vi "RT Driver VI.vi"(6 "Device Clock":string, 9 "Device Inputs FIFO":refnum<k33>, 10 "Device Outputs FIFO":refnum<k33>, 11 "Device Reference":T4 format="%.0x") -> ()   [LabVIEW 2017, in "ALMA_10201-10401_O2SensorSim Engine.lvlib"]
uses:
  ALMA_10201-10401_O2SensorSim Engine.lvlib
  <vilib>/NI Veristand/Custom Device API/Custom Device Item Ref.ctl
  Par.ctl
  LambdaType.ctl
  Sensor_used.ctl
  <vilib>/NI Veristand/Custom Device API/Custom Device Channel Type.ctl
  <vilib>/Platform/TimedLoop/XDataNode/timing_clust.ctl
  <vilib>/Platform/TimedLoop/XDataNode/nitl_modes.ctl
  <vilib>/Platform/TimedLoop/XDataNode/wakeup.ctl
  <vilib>/NI Veristand/Custom Device API/Message Response (String).ctl
  <vilib>/NI Veristand/Custom Device API/Message Response (Byte Array).ctl
  <vilib>/NI Veristand/Custom Device API/Get Item Property (String).vi
  <vilib>/SLSC/Initialize Session with Devices.vi
  <vilib>/SLSC/Close Session.vi
  <vilib>/Platform/TimedLoop/XDataNode/XDataNode.xnode
  <vilib>/NI Veristand/Custom Device API/Custom Device API.lvlib
  <vilib>/NI Veristand/Custom Device Tools/Custom Device Utility Library/Custom Device Utility Library.lvlib
  <vilib>/Platform/TimedLoop/XDataNode/XDNodeRunTimeDep.lvlib
  <vilib>/SLSC/SLSC.lvlib
  System Explorer/SLSC CD API/SLSC CD Engine/SLSC CD Engine.lvlib
panel:
  in  "SensorUsed":T1
  out "Device Session":refnum<k21>
  in  "par 2":T2={"Loop time"={"Loop Rate"=0, "Processor"=0}, "COM"={"COM IP"="0.0.0.0", "COM port"=1, "Local port"=0, "Next_IP 1"=0, "Next_IP 2"=0, "Next_IP 3"=0, "Next_IP 4"=0}, "O2Sensor1"={"Lambda"={"LSU4.2 Lambda"=[], "LSU4.2 Ip"=[], "LSU4.9 Lambda"=[], "LSU4.9 Ip"=[], "LZA03 Lambda"=[], "LZA03 Ip"=[], "LZA08 Lambda"=[], "LZA08 Ip"=[], "Custom Lambda"=[], "Custom Ip"=[]}, "Temp"={"LSU4.2 Temp"=[], "LSU4.2 Ohm"=[], "LSU4.9 Temp"=[], "LSU4.9 Ohm"=[], "LZA03 Temp"=[], "LZA03 Ohm"=[], "LZA08 Temp"=[], "LZA08 Ohm"=[], "Custom Temp"=[], "Custom Ohm"=[]}, "Lambda Type"=0, "PID"={"Ki"=0.0, "Kp"=0.0, "Kd"=0.0, "FeedFW"=0.0}}, "O2Sensor2"={"Lambda"={"LSU4.2 Lambda"=[], "LSU4.2 Ip"=[], "LSU4.9 Lambda"=[], "LSU4.9 Ip"=[], "LZA03 Lambda"=[], "LZA03 Ip"=[], "LZA08 Lambda"=[], "LZA08 Ip"=[], "Custom Lambda"=[], "Custom Ip"=[]}, "Temp"={"LSU4.2 Temp"=[], "LSU4.2 Ohm"=[], "LSU4.9 Temp"=[], "LSU4.9 Ohm"=[], "LZA03 Temp"=[], "LZA03 Ohm"=[], "LZA08 Temp"=[], "LZA08 Ohm"=[], "Custom Temp"=[], "Custom Ohm"=[]}, "Lambda Type"=0, "PID"={"Ki"=0.0, "Kp"=0.0, "Kd"=0.0, "FeedFW"=0.0}}, "O2Sensor3"={"Lambda"={"LSU4.2 Lambda"=[], "LSU4.2 Ip"=[], "LSU4.9 Lambda"=[], "LSU4.9 Ip"=[], "LZA03 Lambda"=[], "LZA03 Ip"=[], "LZA08 Lambda"=[], "LZA08 Ip"=[], "Custom Lambda"=[], "Custom Ip"=[]}, "Temp"={"LSU4.2 Temp"=[], "LSU4.2 Ohm"=[], "LSU4.9 Temp"=[], "LSU4.9 Ohm"=[], "LZA03 Temp"=[], "LZA03 Ohm"=[], "LZA08 Temp"=[], "LZA08 Ohm"=[], "Custom Temp"=[], "Custom Ohm"=[]}, "Lambda Type"=0, "PID"={"Ki"=0.0, "Kp"=0.0, "Kd"=0.0, "FeedFW"=0.0}}, "O2Sensor4"={"Lambda"={"LSU4.2 Lambda"=[], "LSU4.2 Ip"=[], "LSU4.9 Lambda"=[], "LSU4.9 Ip"=[], "LZA03 Lambda"=[], "LZA03 Ip"=[], "LZA08 Lambda"=[], "LZA08 Ip"=[], "Custom Lambda"=[], "Custom Ip"=[]}, "Temp"={"LSU4.2 Temp"=[], "LSU4.2 Ohm"=[], "LSU4.9 Temp"=[], "LSU4.9 Ohm"=[], "LZA03 Temp"=[], "LZA03 Ohm"=[], "LZA08 Temp"=[], "LZA08 Ohm"=[], "Custom Temp"=[], "Custom Ohm"=[]}, "Lambda Type"=0, "PID"={"Ki"=0.0, "Kp"=0.0, "Kd"=0.0, "FeedFW"=0.0}}, "Board"=0, "Mode"=enum."SLSC Mode", "vendor.Num"=4141, "product.Num"=0} {"Board" items=["O2Sim_2ch", "O2Sim_4ch"]; "O2Sensor4"."Lambda Type" items=["LSU4.2", "LSU4.9", "LZA03", "LZA08", "Custom", "[mA]"]; "O2Sensor3"."Lambda Type" items=["LSU4.2", "LSU4.9", "LZA03", "LZA08", "Custom", "[mA]"]; "O2Sensor2"."Lambda Type" items=["LSU4.2", "LSU4.9", "LZA03", "LZA08", "Custom", "[mA]"]; "O2Sensor1"."Lambda Type" items=["LSU4.2", "LSU4.9", "LZA03", "LZA08", "Custom", "[mA]"]}
  in  "Initialization Status Notifier":refnum<notifier>
  in  "Status Notifier":refnum<notifier>
  # "Custom Device Template\nv1.0"
  # "Use this template as a starting point for creating a custom device code module. The input controls shown here are specially named controls that the system will use to provide the device loop with data. The controls are not required for the device loop to run. For instance, if the device doesn't produce any output data, then you don't need the Device Outputs FIFO control. If you do use these controls, however, they need to have these exact names to be functional."
  # "The optional status notifier element is used to notify the RT engine of the last state of the custom device, and to indicate the device has completed execution. If this control is not used, a default No Error value is returned to the system when the device finishes execution.\n\nNote: This error state is not checked until the system shuts down. Use an output status channel to send more immediate status values to the system."
  # "This optional input can be used to send the VeriStand Engine the final status of the custom device initalization process. If this control exists on the custom device front panel, the VeriStand Engine will wait for a status update before starting up. If the custom device reports an error, that will abort the execution of the current configuration in the VeriStand Engine.\n\nThis control can be deleted if the custom device does not need to send the initialization status update."
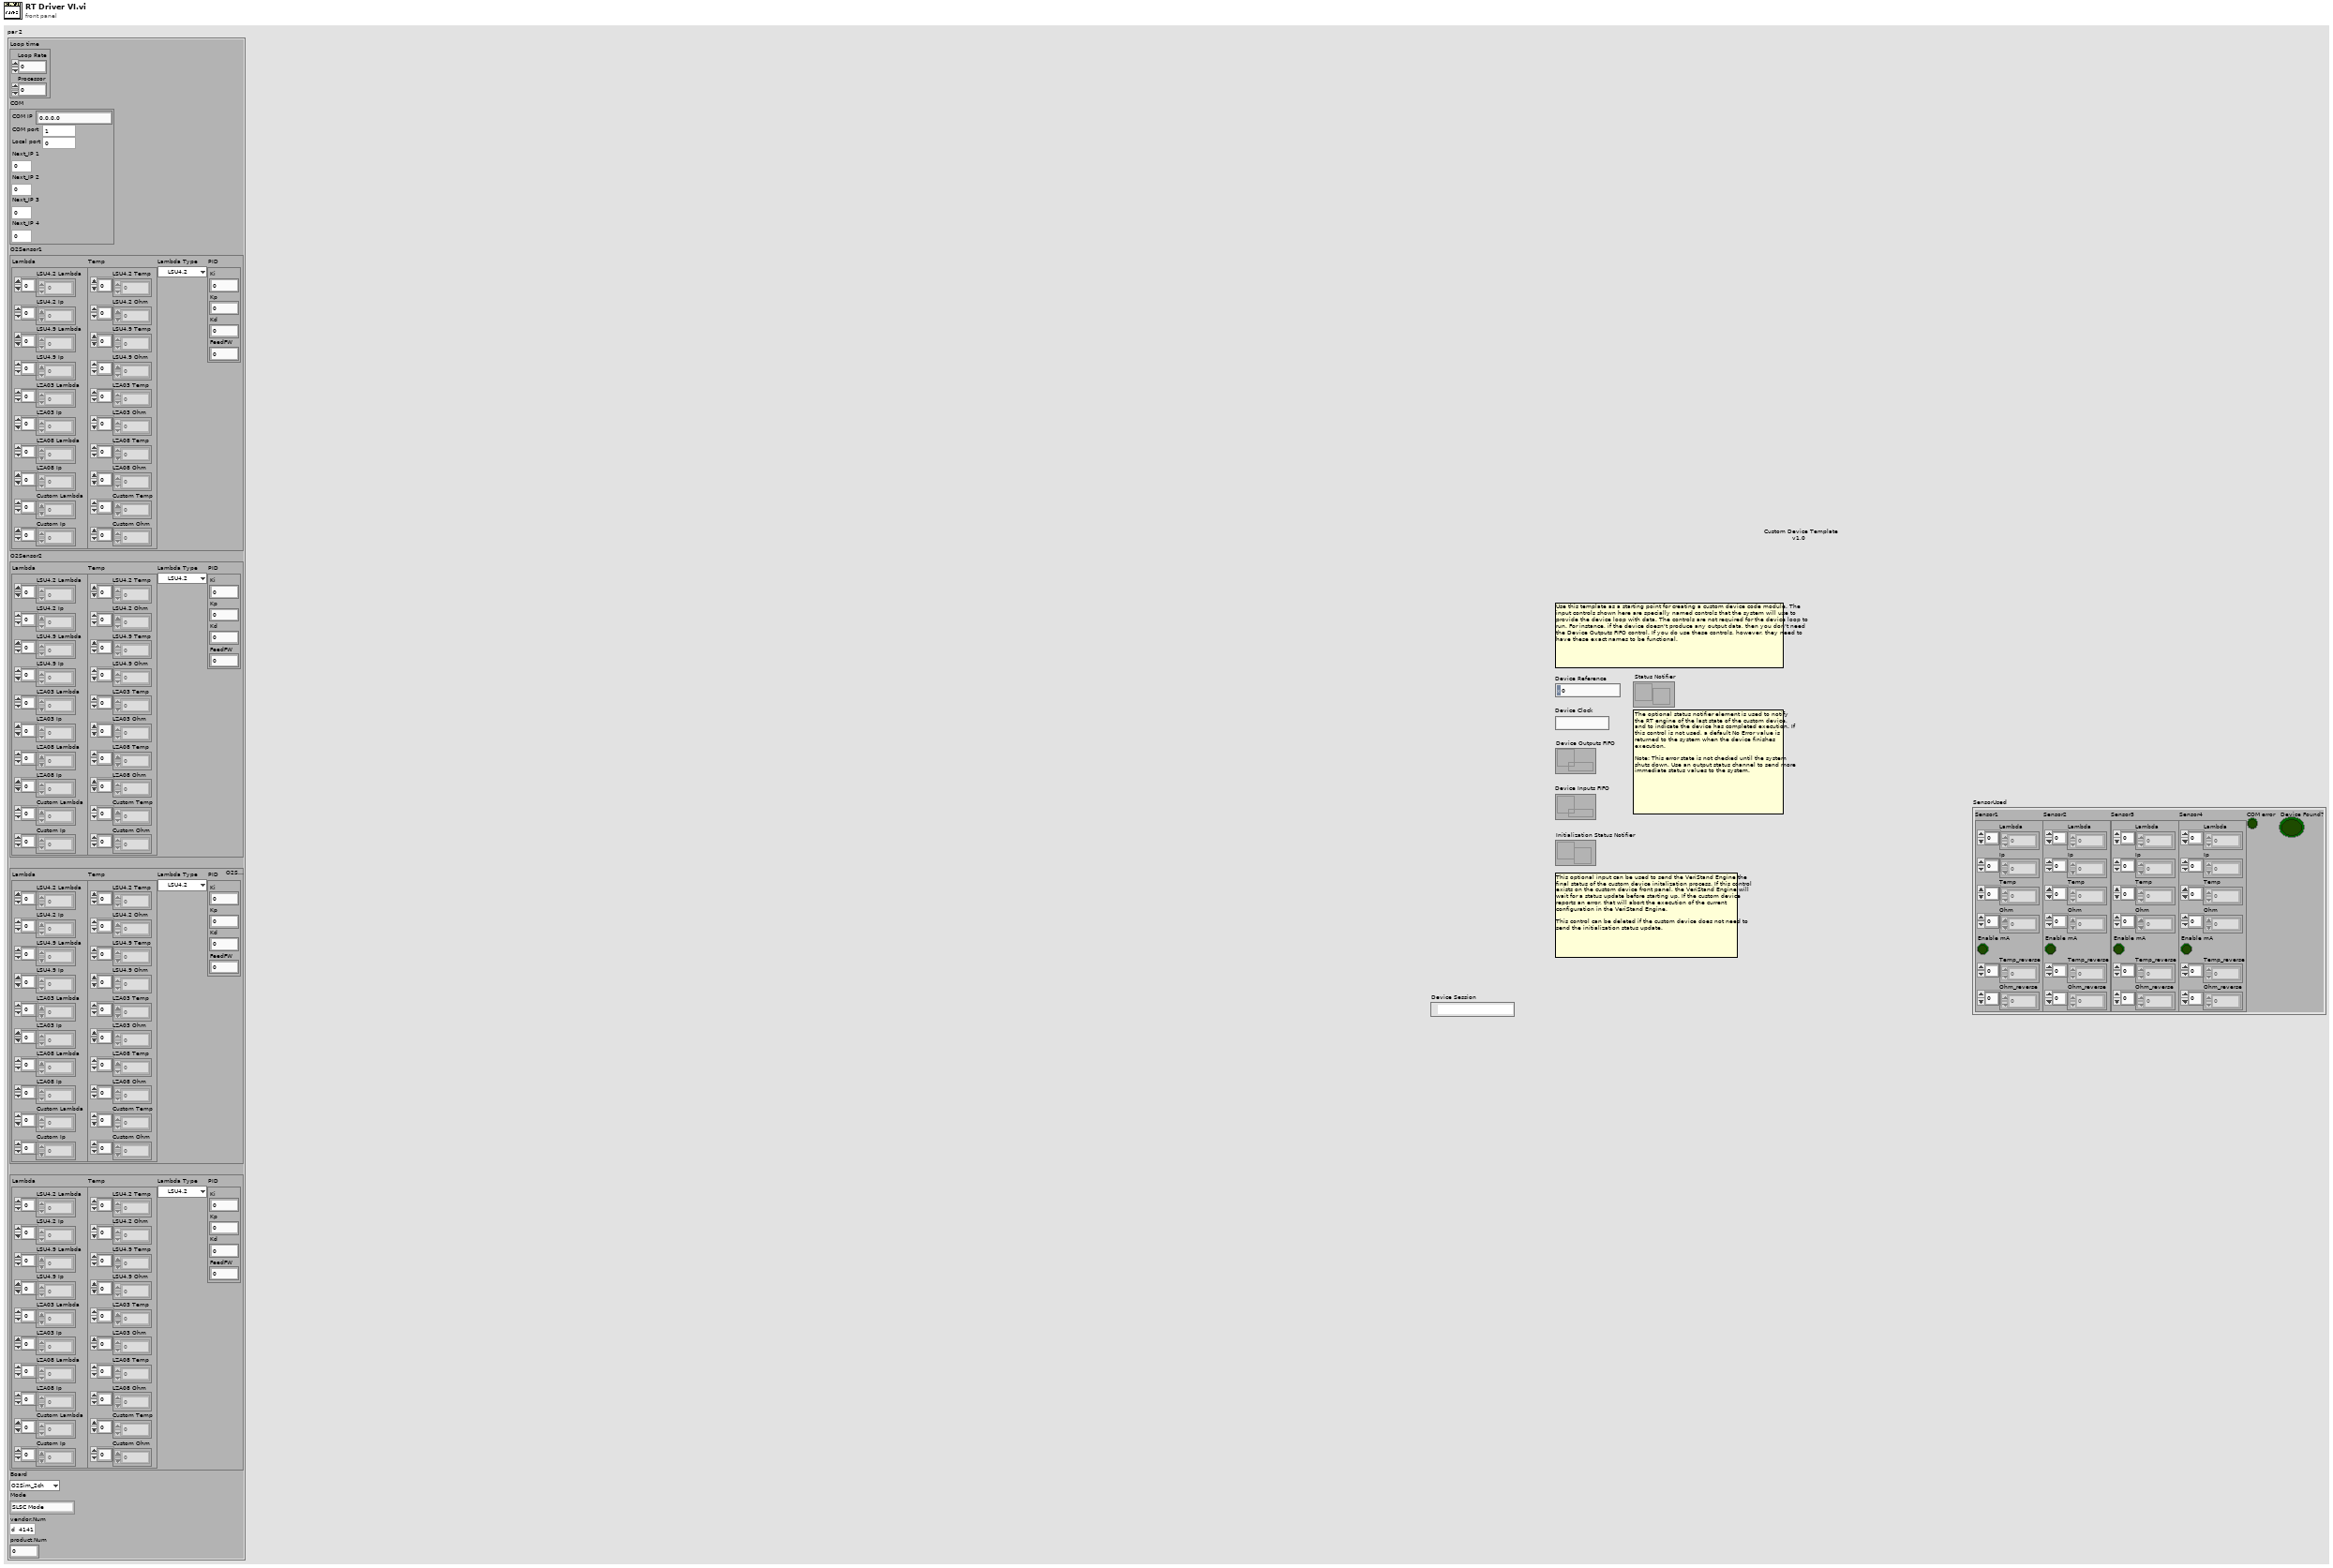
[diagram p1: front panel]
types:
  T1 = typedef "ALMA_10201-10401_O2SensorSim Engine.lvlib/Sensor_used.ctl" = cluster{"Sensor1":cluster{"Lambda":dbl[], "Ip":dbl[], "Temp":dbl[], "Ohm":dbl[], "Enable mA":bool, "Temp_reverse":dbl[], "Ohm_reverse":dbl[]}, "Sensor2":cluster{"Lambda":dbl[], "Ip":dbl[], "Temp":dbl[], "Ohm":dbl[], "Enable mA":bool, "Temp_reverse":dbl[], "Ohm_reverse":dbl[]}, "Sensor3":cluster{"Lambda":dbl[], "Ip":dbl[], "Temp":dbl[], "Ohm":dbl[], "Enable mA":bool, "Temp_reverse":dbl[], "Ohm_reverse":dbl[]}, "Sensor4":cluster{"Lambda":dbl[], "Ip":dbl[], "Temp":dbl[], "Ohm":dbl[], "Enable mA":bool, "Temp_reverse":dbl[], "Ohm_reverse":dbl[]}, "COM error":bool, "Device Found?":bool}
  T2 = typedef "Par.ctl" = cluster{"Loop time":cluster{"Loop Rate":i64, "Processor":i32}, "COM":cluster{"COM IP":string, "COM port":u64, "Local port":u64, "Next_IP 1":u32, "Next_IP 2":u32, "Next_IP 3":u32, "Next_IP 4":u32}, "O2Sensor1":cluster{"Lambda":cluster{"LSU4.2 Lambda":dbl[], "LSU4.2 Ip":dbl[], "LSU4.9 Lambda":dbl[], "LSU4.9 Ip":dbl[], "LZA03 Lambda":dbl[], "LZA03 Ip":dbl[], "LZA08 Lambda":dbl[], "LZA08 Ip":dbl[], "Custom Lambda":dbl[], "Custom Ip":dbl[]}, "Temp":cluster{"LSU4.2 Temp":dbl[], "LSU4.2 Ohm":dbl[], "LSU4.9 Temp":dbl[], "LSU4.9 Ohm":dbl[], "LZA03 Temp":dbl[], "LZA03 Ohm":dbl[], "LZA08 Temp":dbl[], "LZA08 Ohm":dbl[], "Custom Temp":dbl[], "Custom Ohm":dbl[]}, "Lambda Type":T3, "PID":cluster{"Ki":dbl, "Kp":dbl, "Kd":dbl, "FeedFW":dbl}}, "O2Sensor2":cluster{"Lambda":cluster{"LSU4.2 Lambda":dbl[], "LSU4.2 Ip":dbl[], "LSU4.9 Lambda":dbl[], "LSU4.9 Ip":dbl[], "LZA03 Lambda":dbl[], "LZA03 Ip":dbl[], "LZA08 Lambda":dbl[], "LZA08 Ip":dbl[], "Custom Lambda":dbl[], "Custom Ip":dbl[]}, "Temp":cluster{"LSU4.2 Temp":dbl[], "LSU4.2 Ohm":dbl[], "LSU4.9 Temp":dbl[], "LSU4.9 Ohm":dbl[], "LZA03 Temp":dbl[], "LZA03 Ohm":dbl[], "LZA08 Temp":dbl[], "LZA08 Ohm":dbl[], "Custom Temp":dbl[], "Custom Ohm":dbl[]}, "Lambda Type":T3, "PID":cluster{"Ki":dbl, "Kp":dbl, "Kd":dbl, "FeedFW":dbl}}, "O2Sensor3":cluster{"Lambda":cluster{"LSU4.2 Lambda":dbl[], "LSU4.2 Ip":dbl[], "LSU4.9 Lambda":dbl[], "LSU4.9 Ip":dbl[], "LZA03 Lambda":dbl[], "LZA03 Ip":dbl[], "LZA08 Lambda":dbl[], "LZA08 Ip":dbl[], "Custom Lambda":dbl[], "Custom Ip":dbl[]}, "Temp":cluster{"LSU4.2 Temp":dbl[], "LSU4.2 Ohm":dbl[], "LSU4.9 Temp":dbl[], "LSU4.9 Ohm":dbl[], "LZA03 Temp":dbl[], "LZA03 Ohm":dbl[], "LZA08 Temp":dbl[], "LZA08 Ohm":dbl[], "Custom Temp":dbl[], "Custom Ohm":dbl[]}, "Lambda Type":T3, "PID":cluster{"Ki":dbl, "Kp":dbl, "Kd":dbl, "FeedFW":dbl}}, "O2Sensor4":cluster{"Lambda":cluster{"LSU4.2 Lambda":dbl[], "LSU4.2 Ip":dbl[], "LSU4.9 Lambda":dbl[], "LSU4.9 Ip":dbl[], "LZA03 Lambda":dbl[], "LZA03 Ip":dbl[], "LZA08 Lambda":dbl[], "LZA08 Ip":dbl[], "Custom Lambda":dbl[], "Custom Ip":dbl[]}, "Temp":cluster{"LSU4.2 Temp":dbl[], "LSU4.2 Ohm":dbl[], "LSU4.9 Temp":dbl[], "LSU4.9 Ohm":dbl[], "LZA03 Temp":dbl[], "LZA03 Ohm":dbl[], "LZA08 Temp":dbl[], "LZA08 Ohm":dbl[], "Custom Temp":dbl[], "Custom Ohm":dbl[]}, "Lambda Type":T3, "PID":cluster{"Ki":dbl, "Kp":dbl, "Kd":dbl, "FeedFW":dbl}}, "Board":u16, "Mode":enum16{"SLSC Mode", "ANALOG Mode"}, "vendor.Num":u32, "product.Num":u32}
  T3 = typedef "LambdaType.ctl" = u16
  T4 = typedef "Custom Device API.lvlib/Custom Device Item Ref.ctl" = u64
  T5 = typedef "Custom Device API.lvlib/Custom Device Channel Type.ctl" = enum16{"Input", "Output"}
  T6 = cluster{"Lambda":cluster{"LSU4.2 Lambda":dbl[], "LSU4.2 Ip":dbl[], "LSU4.9 Lambda":dbl[], "LSU4.9 Ip":dbl[], "LZA03 Lambda":dbl[], "LZA03 Ip":dbl[], "LZA08 Lambda":dbl[], "LZA08 Ip":dbl[], "Custom Lambda":dbl[], "Custom Ip":dbl[]}, "Temp":cluster{"LSU4.2 Temp":dbl[], "LSU4.2 Ohm":dbl[], "LSU4.9 Temp":dbl[], "LSU4.9 Ohm":dbl[], "LZA03 Temp":dbl[], "LZA03 Ohm":dbl[], "LZA08 Temp":dbl[], "LZA08 Ohm":dbl[], "Custom Temp":dbl[], "Custom Ohm":dbl[]}, "Lambda Type":T3, "PID":cluster{"Ki":dbl, "Kp":dbl, "Kd":dbl, "FeedFW":dbl}}
  T7 = cluster{"Lambda":cluster{"LSU4.2 Lambda":dbl[], "LSU4.2 Ip":dbl[], "LSU4.9 Lambda":dbl[], "LSU4.9 Ip":dbl[], "LZA03 Lambda":dbl[], "LZA03 Ip":dbl[], "LZA08 Lambda":dbl[], "LZA08 Ip":dbl[], "Custom Lambda":dbl[], "Custom Ip":dbl[]}, "Temp":cluster{"LSU4.2 Temp":dbl[], "LSU4.2 Ohm":dbl[], "LSU4.9 Temp":dbl[], "LSU4.9 Ohm":dbl[], "LZA03 Temp":dbl[], "LZA03 Ohm":dbl[], "LZA08 Temp":dbl[], "LZA08 Ohm":dbl[], "Custom Temp":dbl[], "Custom Ohm":dbl[]}, "Lambda Type":T3, "PID":cluster{"Ki":dbl, "Kp":dbl, "Kd":dbl, "FeedFW":dbl}}[]
  T8 = typedef "Custom Device API.lvlib/Custom Device Engine Event Ref.ctl" = refnum<event-registration>
  T9 = cluster{"Custom Lambda":dbl[], "Custom Lambda":dbl[], "Custom Lambda":dbl[], "Custom Lambda":dbl[], bool, "Custom Lambda":dbl[], "Custom Lambda":dbl[]}
  T10 = typedef "XDNodeRunTimeDep.lvlib/timing_clust.ctl" = cluster{"Expected End [f-1]":u64, "Actual End [f-1]":u64, "Finished Late? [f-1]":bool, "Expected End [i-1]":u64, "Actual End [i-1]":u64, "Finished Late? [i-1]":bool, "Expected Start [i]":u64, "Actual Start [i]":u64, "Expected Start [f]":u64, "Actual Start [f]":u64, "Source Name":string, "Structure Name":string, "Period":i64, "Deadline":i64, "Offset":i64, "Start":i64, "Priority":i32, "Timeout":i32, "Mode":T11, "Wakeup Reason":T12, "Error":errorcluster, "Source Type":string, "Secondary Source Type":string, "Global End Time":u64, "Global Start Time":u64, "Frame Duration":u64, "Iteration Duration":u64, "Assigned CPU":i32, "I/O Scan Engine Mode":u32}
  T11 = typedef "XDNodeRunTimeDep.lvlib/nitl_modes.ctl" = enum32{"No Change", "Process missed periods, maintain original phase", "Discard missed periods, maintain original phase", "Process missed periods, ignore original phase", "Discard missed periods, ignore original phase"}
  T12 = typedef "XDNodeRunTimeDep.lvlib/wakeup.ctl" = enum32{"Normal", "Aborted", "Asynchronous wakeup", "Timing source error", "Timed loop error", "Timeout"}
  T13 = typedef "Custom Device API.lvlib/Message Response (String).ctl" = cluster{"Response":string, "Error":errorcluster}
  T14 = typedef "Custom Device API.lvlib/Message Response (Byte Array).ctl" = cluster{"Response":u8[], "Error":errorcluster}
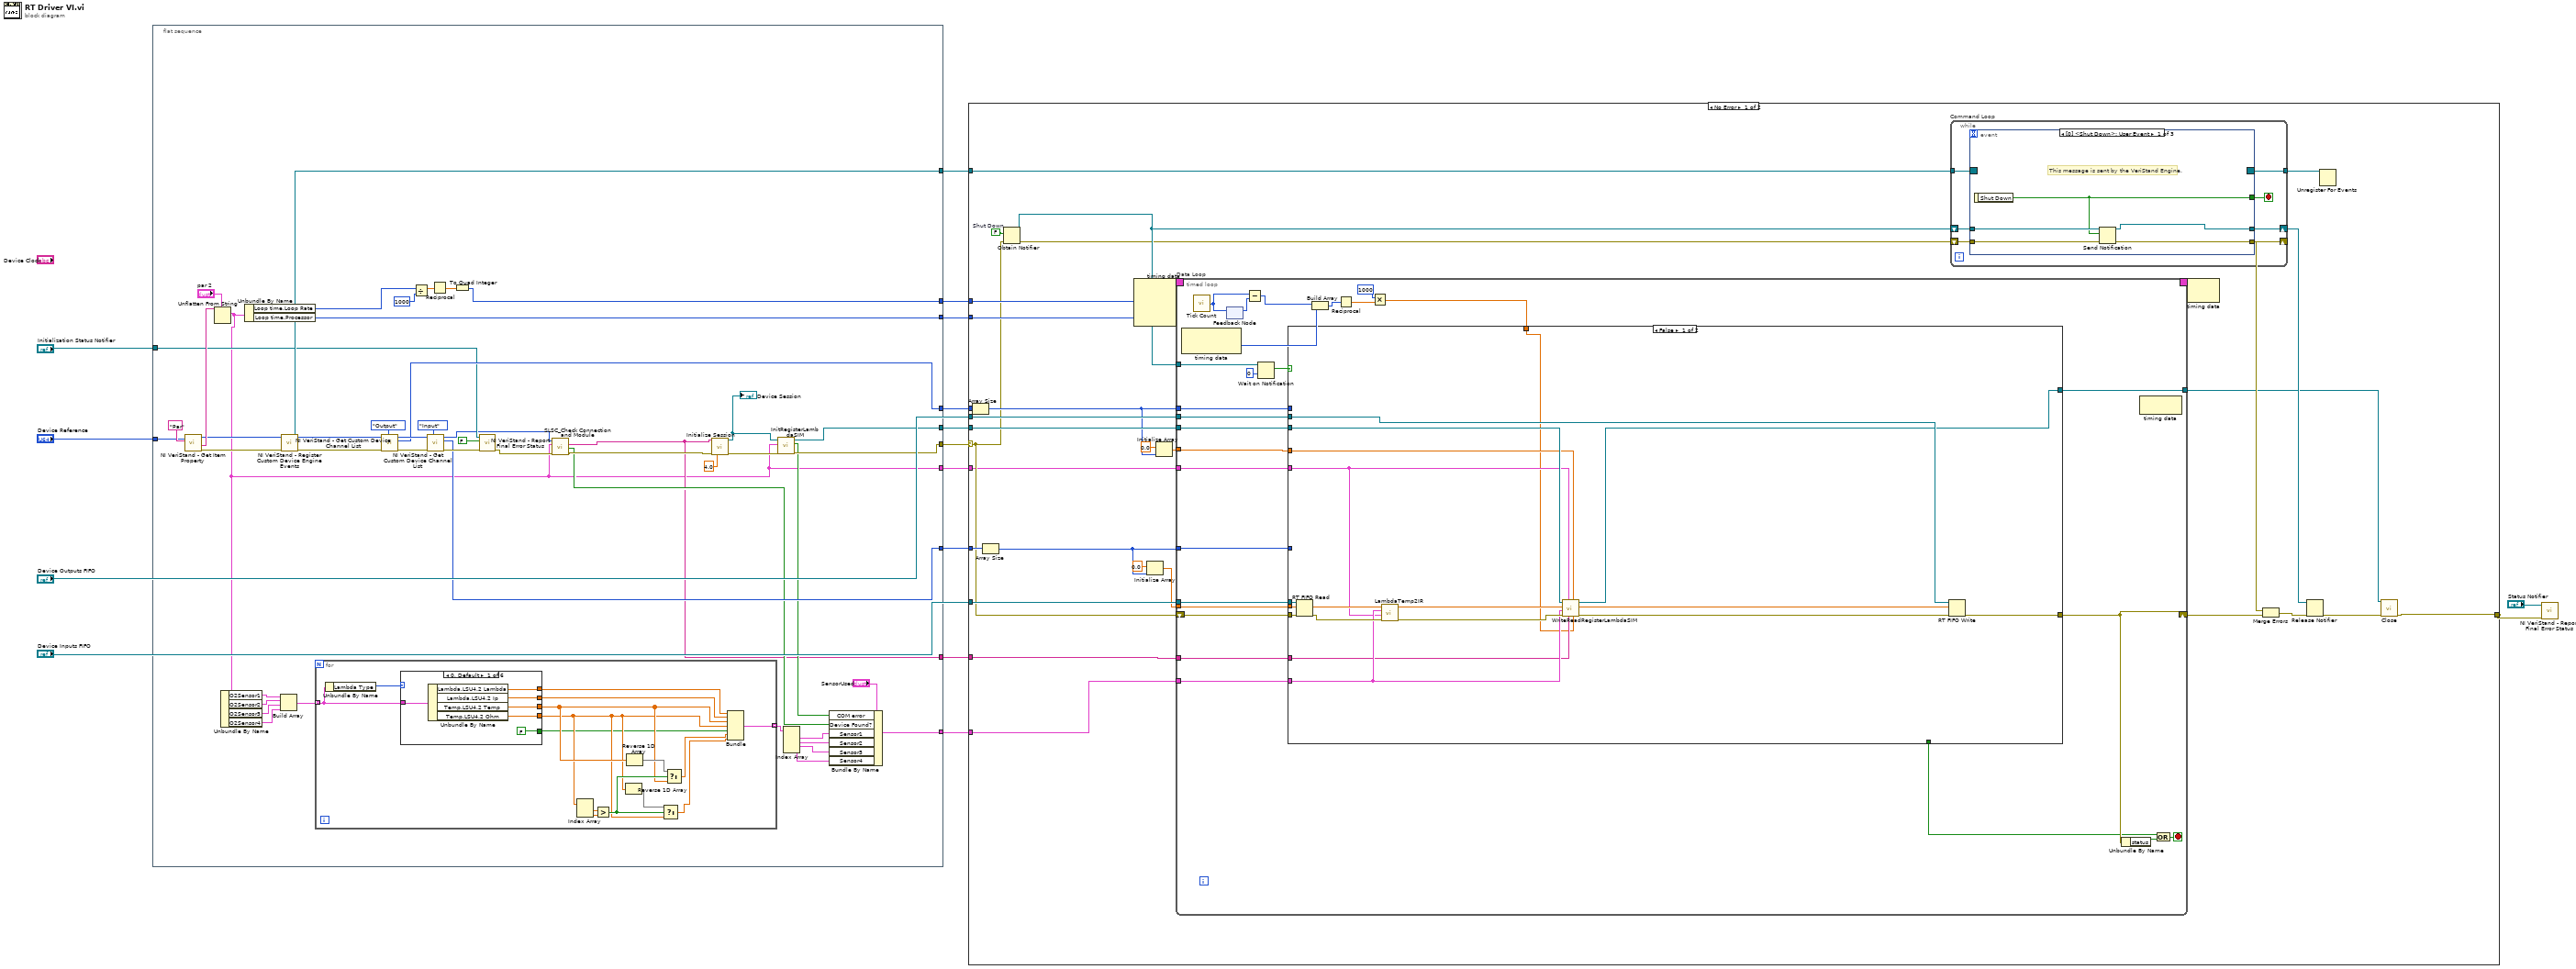
[diagram p0: block diagram]
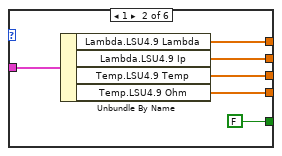
[diagram p2: hidden frame]
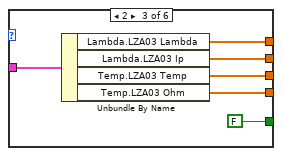
[diagram p3: hidden frame]
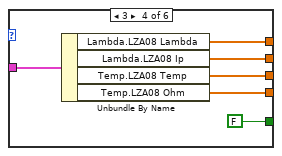
[diagram p4: hidden frame]
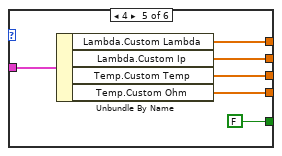
[diagram p5: hidden frame]
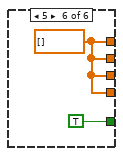
[diagram p6: hidden frame]
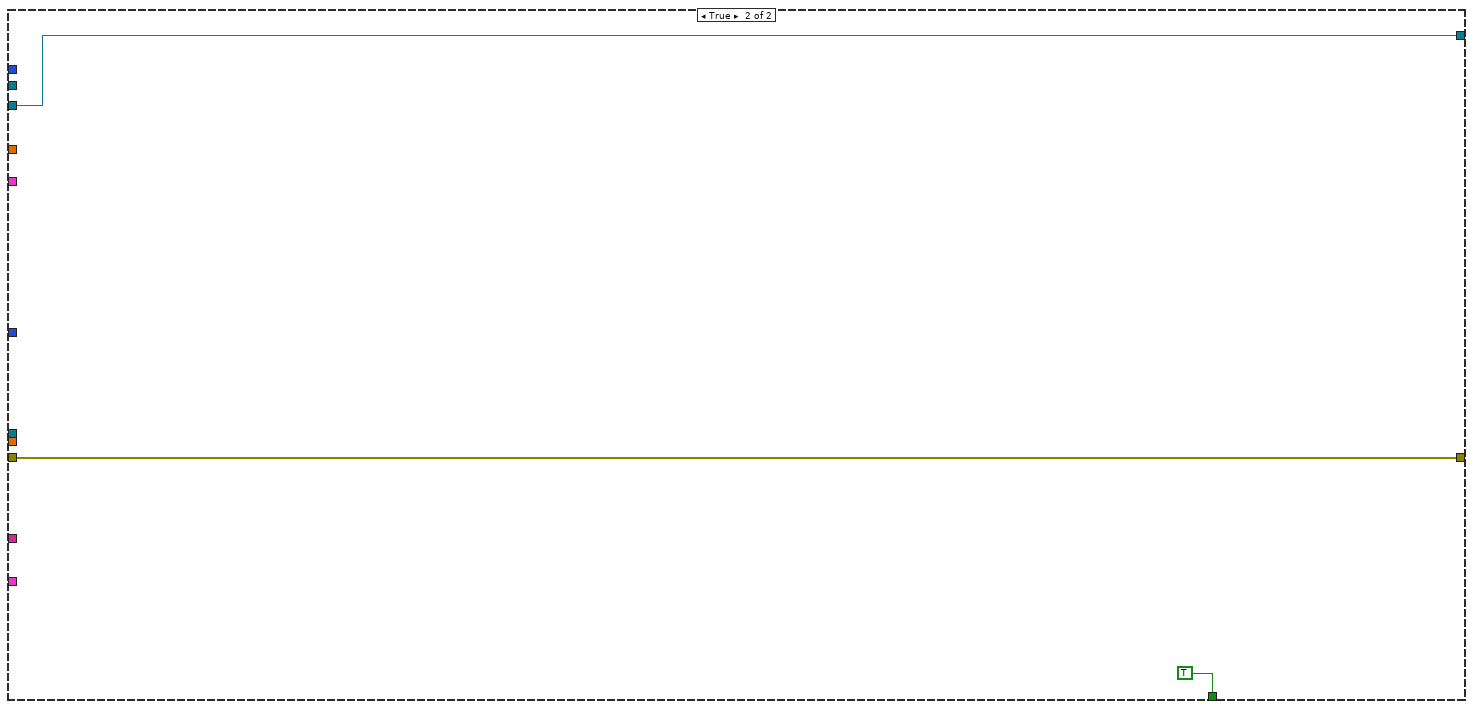
[diagram p7: hidden frame]
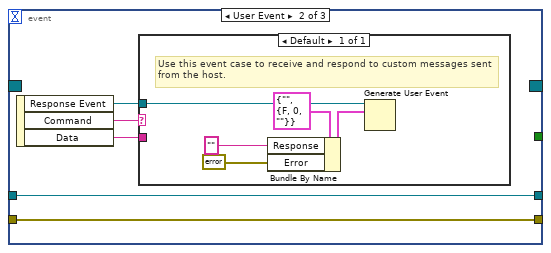
[diagram p8: hidden frame]
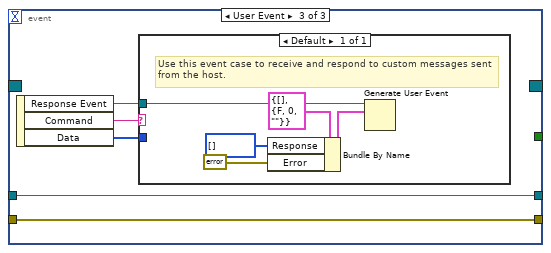
[diagram p9: hidden frame]
diagram:
  n1 = flat-sequence {
    tunnel: [w58] -> w15
    tunnel: [w57] -> w14
    tunnel: [w56] -> w13
    tunnel: [w17] -> w12
    tunnel: [w50] -> w11
    tunnel: "Initialization Status Notifier" -> [w47]
    tunnel: "Device Reference" -> [w46]
    tunnel: [w27] -> w5
    tunnel: [w45] -> w4
    tunnel: [w22] -> w3
    tunnel: [w32] -> w2
    tunnel: [w23] -> w1
    frame #0 {
      n2 = call-poly <vilib>:"NI VeriStand - Get Item Property.vi"("Property Name"="Par", "Item Ref in"=w46) -> ("error out"=w49:errorcluster, "Value"=w52:string, "Item Ref out"=w51:T4)  [unwired: 6 in, 1 out]
      n3 = Unflatten From String(type="par 2", binary string=w52) -> (value=w22:T2)  [unwired: 3 in, 2 out]
      n4 = Unbundle By Name(w22) -> ("O2Sensor1"=w42:T6, "O2Sensor2"=w41:T6, "O2Sensor3"=w40:T6, "O2Sensor4"=w39:T6)
      n5 = Unbundle By Name(w22) -> ("Loop time.Loop Rate"=w19:i64, "Loop time.Processor"=w50:i32)
      n6 = Build Array(w42, w41, w40, w39) -> (w38:T7)
      n7 = call <vilib>:"NI VeriStand - Register Custom Device Engine Events.vi"("error in (no error)"=w49, "Device Ref in"=w51) -> ("error out"=w64:errorcluster, "Custom Device Engine Event Ref"=w56:T8, "Device Ref out"=w55:T4)  [unwired: 7 in]
      n8 = for {
        tunnel: w38 -> [w66] mode=indexing
        tunnel: [w67] -> w37 mode=indexing
        n9 = Unbundle By Name(w66) -> ("Lambda Type"=w65:T3)
        n10 = case shown="0, Default" w65 {
          tunnel: w66 -> [w85 w91 w97 w103 w109 _]
          tunnel: [w83 w89 w95 w101 w107 w110] -> w74
          tunnel: [w82 w88 w94 w100 w106 w110] -> w73
          tunnel: [FALSE FALSE FALSE FALSE FALSE TRUE] -> w70
          tunnel: [w81 w87 w93 w99 w105 w110] -> w72
          tunnel: [w80 w86 w92 w98 w104 w110] -> w71
          frame 0, Default {
            n11 = Unbundle By Name(w85) -> ("Lambda.LSU4.2 Lambda"=w83:dbl[], "Lambda.LSU4.2 Ip"=w82:dbl[], "Temp.LSU4.2 Temp"=w81:dbl[], "Temp.LSU4.2 Ohm"=w80:dbl[])
          }
          frame 1 {
            n12 = Unbundle By Name(w91) -> ("Lambda.LSU4.9 Lambda"=w89:dbl[], "Lambda.LSU4.9 Ip"=w88:dbl[], "Temp.LSU4.9 Temp"=w87:dbl[], "Temp.LSU4.9 Ohm"=w86:dbl[])
          }
          frame 2 {
            n13 = Unbundle By Name(w97) -> ("Lambda.LZA03 Lambda"=w95:dbl[], "Lambda.LZA03 Ip"=w94:dbl[], "Temp.LZA03 Temp"=w93:dbl[], "Temp.LZA03 Ohm"=w92:dbl[])
          }
          frame 3 {
            n14 = Unbundle By Name(w103) -> ("Lambda.LZA08 Lambda"=w101:dbl[], "Lambda.LZA08 Ip"=w100:dbl[], "Temp.LZA08 Temp"=w99:dbl[], "Temp.LZA08 Ohm"=w98:dbl[])
          }
          frame 4 {
            n15 = Unbundle By Name(w109) -> ("Lambda.Custom Lambda"=w107:dbl[], "Lambda.Custom Ip"=w106:dbl[], "Temp.Custom Temp"=w105:dbl[], "Temp.Custom Ohm"=w104:dbl[])
          }
          frame 5 {
            w110 = dbl[] [] ("Custom Lambda")
          }
        }
        n16 = Index Array(array=w71) -> (element #1=w77:dbl, element #2=w78:dbl)  [unwired: 2 in]
        n17 = Greater?(x=w77, y=w78) -> (0:w75:bool)
        n18 = Reverse 1D Array(array=w71) -> (reversed array=w79:dbl[])
        n19 = Reverse 1D Array(array=w72) -> (reversed array=w76:dbl[])
        n20 = Select(t=w79, s=w75, f=w71) -> (s? t:f=w68:dbl[])
        n21 = Select(t=w76, s=w75, f=w72) -> (s? t:f=w69:dbl[])
        n22 = Bundle("Custom Lambda"=w74, "Custom Lambda"=w73, "Custom Lambda"=w72, "Custom Lambda"=w71, w70, "Custom Lambda"=w69, "Custom Lambda"=w68) -> (w67:T9)  [unwired: 1 in]
      }
      n23 = call <vilib>:"NI VeriStand - Get Custom Device Channel List.vi"("Channel Type"=Custom_Device_Channel_Type."Output", "error in (no error)"=w64, "Device Ref in"=w55) -> ("error out"=w60:errorcluster, "Specified Channel Ref List"=w57:T4[], "Device Ref out"=w61:T4)  [unwired: 6 out]
      n24 = Divide(x=w19, y=i64 1000 ("upper limit")) -> (x/y=w21:dbl)
      n25 = call <vilib>:"NI VeriStand - Get Custom Device Channel List.vi"("Channel Type"=Custom_Device_Channel_Type."Input", "error in (no error)"=w60, "Device Ref in"=w61) -> ("error out"=w63:errorcluster, "Specified Channel Ref List"=w58:T4[], "Device Ref out"=w24:T4)  [unwired: 6 out]
      n26 = Reciprocal(x=w21) -> (1/x=w18:dbl)
      n27 = To Quad Integer(1:w18) -> (0:w17:i64)
      n28 = call <vilib>:"NI VeriStand - Report Final Error Status.vi"("error in (no error)"=w63, "Filter FIFO & Shutdown Errors (T)"=FALSE ("Filter FIFO Errors (T)"), "Status Notifier"=w47) -> ("error out"=w25:errorcluster)  [unwired: 8 out]
      n29 = call "SLSC_Check Connection and Module.vi"("error in (no error)"=w25, "par"=w22, "Device Reference"=w24) -> ("error out"=w29:errorcluster, "Device Found?"=w28:bool, "SLSC IP"=w23:string)  [unwired: 3 in, 3 out]
      n30 = call-poly <vilib>:"Initialize Session.vi"("devices"=w23, "error in (no error)"=w29, "connect timeout (60 sec)"=4.0) -> ("session out"=w31:refnum<k21>, "error out"=w30:errorcluster)  [unwired: 11 in]
      "Device Session" <- w31
      n31 = call "InitRegisterLambdaSIM.vi"("error in"=w30, "value"=w22, "session in"=w31) -> ("error out"=w27:errorcluster, "COM error"=w26:bool, "session out"=w45:refnum<k21>)  [unwired: 6 in]
      n32 = Index Array(array=w37) -> (element #1=w36:T9, element #2=w35:T9, element #3=w34:T9, element #4=w33:T9)  [unwired: 4 in]
      n33 = Bundle By Name(cluster="SensorUsed", "COM error"=w26, "Device Found?"=w28, "Sensor1"=w36, "Sensor2"=w35, "Sensor3"=w34, "Sensor4"=w33) -> (w32:T1)
    }
  }
  n34 = case shown="No Error" w5 {
    selector: w5 -> [w116 w231]
    tunnel: "Device Outputs FIFO" -> [w142 _]
    tunnel: "Device Inputs FIFO" -> [w141 _]
    tunnel: w15 -> [w139 _]
    tunnel: w14 -> [w138 _]
    tunnel: w13 -> [w137 _]
    tunnel: [w124 w231] -> w7
    tunnel: w12 -> [w118 _]
    tunnel: w11 -> [w129 _]
    tunnel: w3 -> [w113 _]
    tunnel: w4 -> [w127 _]
    tunnel: w2 -> [w125 _]
    tunnel: w1 -> [w119 _]
    frame No Error {
      w136 = FALSE  # Shut Down
      n35 = Array Size(array=w138) -> (size(s)=w122:i32)
      n36 = Array Size(array=w139) -> (size(s)=w128:i32)
      n37 = Obtain Notifier(notification data type=w136, error in (no error)=w116) -> (notifier out=w134:refnum<notifier>, error out=w112:errorcluster)  [unwired: 2 in, 1 out]
      n38 = node-c288(w118, w129) -> (w131:T10)  [unwired: 2 in]
      n39 = Initialize Array(0.0 ("element"), w128) -> (w117:dbl[])
      n40 = Initialize Array(0.0 ("element"), w122) -> (w121:dbl[])
      n41 = timed-loop "Data Loop" {
        shift-right: [w163] -> w120
        shift-left: w116 -> [w169]
        tunnel: w122 -> [w166]
        tunnel: w142 -> [w168]
        tunnel: w141 -> [w167]
        tunnel: w128 -> [w165]
        tunnel: w134 -> [w162]
        timing: w131 -> [_]
        timing-out: [_] -> w130
        tunnel: w113 -> [w157]
        tunnel: w127 -> [w152]
        tunnel: [w156] -> w126
        tunnel: w125 -> [w155]
        tunnel: w117 -> [w153]
        tunnel: w121 -> [w154]
        tunnel: w119 -> [w151]
        stop <- w158 stop-if-true
        n42 = node-c288() -> (w150:i64)  [unwired: 1 in, 1 out]
        n43 = call "Tick Count"() -> ("Tick Count(mSec)"=w145:u32)
        n44 = feedback-in #1(w145) -> ()
        n45 = feedback #1() -> (w144:u32)  [unwired: 1 in]
        n46 = Subtract(x=w145, y=w144) -> (x-y=w143:u32)
        n47 = Wait on Notification(notifier=w162, timeout in ms (-1)=0) -> (notification=w161:bool)  [unwired: 2 in, 3 out]
        n48 = Build Array(w143, w150) -> (w148:i64[])
        n49 = Reciprocal(x=w148) -> (1/x=w147:dbl[])
        n50 = Multiply(x=i64 1000 ("Period"), y=w147) -> (x*y=w146:dbl[])
        n51 = case shown="False" w161 {
          tunnel: w169 -> [w190 w191]
          tunnel: w153 -> [w189 _]
          tunnel: w168 -> [w188 _]
          tunnel: w167 -> [w187 _]
          tunnel: w166 -> [_ _]
          tunnel: w165 -> [_ _]
          tunnel: [w186 w191] -> w163
          tunnel: [_ TRUE] -> w159
          tunnel: w157 -> [w176 _]
          tunnel: w152 -> [w185 w193]
          tunnel: [w181 w193] -> w156
          tunnel: w155 -> [w179 _]
          tunnel: w154 -> [w175 _]
          tunnel: w151 -> [w174 _]
          tunnel: w146 -> [w173 _]
          frame False {
            n52 = RT FIFO Read(0:w187, 1:w189, 3:w190) -> (9:w184:dbl[], 11:w183:errorcluster)  [unwired: 4 out]
            n53 = call "LambdaTemp2IR.vi"("error constant"=w183, "par 3"=w176, "SensorUsed"=w179, "VS control"=w184) -> ("error constant out"=w182:errorcluster, "VS control out"=w180:dbl[])  [unwired: 6 in]
            n54 = call "WriteReadRegisterLambdaSIM.vi"("period"=w173, "VS feedback"=w175, "devices 2"=w174, "par 3"=w176, "error in"=w182, "SensorUsed"=w179, "VS Control"=w180, "session in"=w185) -> ("error out"=w177:errorcluster, "VS feedback"=w178:dbl[], "session out"=w181:refnum<k21>)  [unwired: 1 in]
            n55 = RT FIFO Write(0:w188, 1:w178, 3:w177) -> (11:w186:errorcluster)  [unwired: 1 in, 4 out]
          }
          frame True {
          }
        }
        n56 = Unbundle By Name(w163) -> ("status"=w160:bool)
        n57 = node-c288() -> ()  [unwired: 1 in, 1 out]
        n58 = Compound Arithmetic op=OR(w159, w160) -> (w158:bool)
      }
      n59 = while "Command Loop" {
        tunnel: w137 -> [w205]
        tunnel: [w204] -> w135
        shift-right: [w201] -> w133
        shift-left: w134 -> [w202]
        shift-right: [w199] -> w132
        shift-left: w112 -> [w200]
        stop <- w203 stop-if-true
        n60 = event shown="[0] <Shut Down>: User Event" {
          selector: w205 -> [_ _ _]
          dyn-events: [_ _ _] -> w204
          timeout: _ -> [_ _ _]
          tunnel: [w207 _ _] -> w203
          tunnel: w202 -> [w209 w213 w223]
          tunnel: [w210 w213 w223] -> w201
          tunnel: w200 -> [w208 w211 w221]
          tunnel: [w206 w211 w221] -> w199
          event User Event {
            # "This message is sent by the VeriStand Engine."
            n61 = event-data() -> ("Shut Down"=w207:bool)  [unwired: 1 in]
            n62 = Send Notification(notification=w207, notifier=w209, error in (no error)=w208) -> (notifier out=w210:refnum<notifier>, error out=w206:errorcluster)
          }
          event User Event {
            n63 = event-data() -> ("Response Event"=w212:refnum<user-event>, "Command"=w215:string, "Data"=w214:string)  [unwired: 1 in]
            n64 = case shown="Default" w215 {
              tunnel: w214 -> [_]
              tunnel: w212 -> [w220]
              frame Default {
                # "Use this event case to receive and respond to custom messages sent from the host."
                n65 = Bundle By Name(cluster=T13 {"Response"="", "Error"={"status"=FALSE, "code"=0, "source"=""}} ("event data"), "Response"="", "Error"=errorcluster {"status"=FALSE, "code"=0, "source"=""}) -> (w218:T13)
                n66 = Generate User Event(user event=w220, event data cluster=w218) -> ()  [unwired: 2 in, 2 out]
              }
            }
          }
          event User Event {
            n67 = event-data() -> ("Response Event"=w222:refnum<user-event>, "Command"=w225:string, "Data"=w224:u8[])  [unwired: 1 in]
            n68 = case shown="Default" w225 {
              tunnel: w224 -> [_]
              tunnel: w222 -> [w230]
              frame Default {
                # "Use this event case to receive and respond to custom messages sent from the host."
                n69 = Bundle By Name(cluster=T14 {"Response"=[], "Error"={"status"=FALSE, "code"=0, "source"=""}} ("event data"), "Response"=u8[] [], "Error"=errorcluster {"status"=FALSE, "code"=0, "source"=""}) -> (w227:T14)
                n70 = Generate User Event(user event=w230, event data cluster=w227) -> ()  [unwired: 2 in, 2 out]
              }
            }
          }
        }
      }
      n71 = node-c288(w130) -> ()  [unwired: 1 out]
      n72 = Merge Errors(w132, w120) -> (w115:errorcluster)
      n73 = Release Notifier(notifier=w133, error in (no error)=w115) -> (error out=w114:errorcluster)  [unwired: 1 in, 2 out]
      n74 = Unregister For Events(event registration refnum=w135) -> ()  [unwired: 1 in, 1 out]
      n75 = call-poly <vilib>:"Close.vi"("session in"=w126, "error in (no error)"=w114) -> ("error out"=w124:errorcluster)  [unwired: 13 in]
    }
    frame Error {
    }
  }
  n76 = call <vilib>:"NI VeriStand - Report Final Error Status.vi"("error in (no error)"=w7, "Status Notifier"="Status Notifier") -> ()  [unwired: 1 in, 9 out]
